vi "MegaAnalysis5.vi"() -> ()   [LabVIEW 2016] (continued)
                n2287 = property on="sampling freq" class="DigNum (strict)"() -> ("Value"=w5459:dbl)  [unwired: 2 in, 2 out]
                n2288 = property on="high cutoff" class="DigNum (strict)"() -> ("Value"=w5456:dbl)  [unwired: 2 in, 2 out]
                n2289 = property on="phase" class="DigNum (strict)"() -> ("Value"=w5444:dbl)  [unwired: 2 in, 2 out]
                n2290 = property on="phase" class="DigNum (strict)"() -> ("Value"=w5451:dbl)  [unwired: 2 in, 2 out]
                n2291 = property on="gamma" class="DigNum (strict)"() -> ("Value"=w5443:dbl)  [unwired: 2 in, 2 out]
                n2292 = property on="order" class="DigNum (strict)"() -> ("Value"=w5455:i32)  [unwired: 2 in, 2 out]
                n2293 = property on="poly sub" class="DigNum (strict)"() -> ("Value"=w5458:dbl)  [unwired: 2 in, 2 out]
                n2294 = Bundle("Value"=w5465, "Value"=w5464, "Value"=w5463, "Value"=w5462, "Value"=w5461, "Value"=w5460, "Value"=w5459, "Value"=w5458, "Value"=w5457, "Value"=w5456, "Value"=w5455, "Value"=w5454, "Value"=w5453, "Value"=w5452, "Value"=w5451, "Value"=w5450, "Value"=w5449, "Value"=w5448, "Value"=w5446, "Value"=w5445, "Value"=w5444, "Value"=w5443) -> (w5447:T37)  [unwired: 1 out]
              }
              frame #2 {
                n2295 = property class="Bool (strict)"() -> ("Value"=w5469:bool)  [unwired: 2 in, 2 out]
                n2296 = property on="cut off selection" class="Arr (strict)"() -> ("Value"=w5468:T10)  [unwired: 2 in, 2 out]
                n2297 = property on="window" class="Ring (strict)"() -> ("Value"=w5467:T9)  [unwired: 2 in, 2 out]
                n2298 = Bundle("Value"=w5469, "Value"=w5468, "Value"=w5467) -> (w5466:T38)  [unwired: 1 out]
              }
              frame #3 {
                n2299 = property on="append string onto file name" class="Str"() -> ("Value"=w5473:string)  [unwired: 2 in, 2 out]
                n2300 = property class="Bool (strict)"() -> ("Value"=w5474:bool)  [unwired: 2 in, 2 out]
                n2301 = property class="Bool (strict)"() -> ("Value"=w5472:bool)  [unwired: 2 in, 2 out]
                n2302 = property class="DigNum (strict)"() -> ("Value"=w5471:u8)  [unwired: 2 in, 2 out]
                n2303 = Bundle("Value"=w5474, "Value"=w5473, "Value"=w5472, "Value"=w5471) -> (w5470:T30)  [unwired: 1 out]
              }
              frame #4 {
                n2304 = property on="upper" class="DigNum (strict)"() -> ("Value"=w5478:dbl)  [unwired: 2 in, 2 out]
                n2305 = property class="Bool (strict)"() -> ("Value"=w5479:bool)  [unwired: 2 in, 2 out]
                n2306 = property on="append name" class="Str"() -> ("Value"=w5476:string)  [unwired: 2 in, 2 out]
                n2307 = property on="lower" class="DigNum (strict)"() -> ("Value"=w5477:dbl)  [unwired: 2 in, 2 out]
                n2308 = Bundle("Value"=w5479, "Value"=w5478, "Value"=w5477, "Value"=w5476) -> (w5475:T39)  [unwired: 1 out]
              }
              frame #5 {
                n2309 = Bundle(w5485, w5484, w5483, w5482, w5481) -> (w5480:T40)  [unwired: 1 out]
              }
            }
            n2310 = property class="Ring (strict)"() -> ("Value"=w5436:u16)  [unwired: 2 in, 2 out]
            n2311 = Bundle("Value"=w5436, w5435) -> (w5434:T41)  [unwired: 1 out]
          }
          frame #4 {
            n2312 = stacked-sequence {
              seq-local: [w5491 _ _] -> [_ _ w5504]
              seq-local: [_ w5498 _] -> [_ _ w5503]
              tunnel: [_ _ w5502] -> w5487
              frame #0 {
                n2313 = property on="spectrum type" class="Ring (strict)"() -> ("Value"=w5497:u16)  [unwired: 2 in, 2 out]
                n2314 = property on="interpolate in:" class="Ring (strict)"() -> ("Value"=w5496:u16)  [unwired: 2 in, 2 out]
                n2315 = property on="peak finder threshold" class="DigNum (strict)"() -> ("Value"=w5490:dbl)  [unwired: 2 in, 2 out]
                n2316 = property class="Bool (strict)"() -> ("Value"=w5495:bool)  [unwired: 2 in, 2 out]
                n2317 = property on="width" class="DigNum (strict)"() -> ("Value"=w5489:dbl)  [unwired: 2 in, 2 out]
                n2318 = property on="padding" class="Ring (strict)"() -> ("Value"=w5494:u16)  [unwired: 2 in, 2 out]
                n2319 = property on="truncate spectrum" class="Ring (strict)"() -> ("Value"=w5492:u16)  [unwired: 2 in, 2 out]
                n2320 = property on="Increase spectral density" class="Ring (strict)"() -> ("Value"=w5493:u16)  [unwired: 2 in, 2 out]
                n2321 = Bundle("Value"=w5497, "Value"=w5496, "Value"=w5495, "Value"=w5490, "Value"=w5494, "Value"=w5493, "Value"=w5492, "Value"=w5489) -> (w5491:T42)  [unwired: 1 out]
              }
              frame #1 {
                n2322 = property on="Maximum Entropy M" class="DigNum (strict)"() -> ("Value"=w5500:dbl)  [unwired: 2 in, 2 out]
                n2323 = property on="FT window" class="Ring (strict)"() -> ("Value"=w5501:T9)  [unwired: 2 in, 2 out]
                n2324 = property on="append name" class="Str"() -> ("Value"=w5499:string)  [unwired: 2 in, 2 out]
                n2325 = Bundle("Value"=w5501, "Value"=w5500, "Value"=w5499) -> (w5498:cluster{"Value":T9, "Value":dbl, "Value":string})  [unwired: 1 out]
              }
              frame #2 {
                n2326 = Bundle(w5504, w5503) -> (w5502:T43)  [unwired: 1 out]
              }
            }
            n2327 = property class="Ring (strict)"() -> ("Value"=w5488:u16)  [unwired: 2 in, 2 out]
            n2328 = Bundle("Value"=w5488, w5487) -> (w5486:T44)  [unwired: 1 out]
          }
          frame #5 {
            n2329 = stacked-sequence {
              seq-local: [w5509 _ _] -> [_ _ w5517]
              seq-local: [_ w5514 _] -> [_ _ w5516]
              tunnel: [_ _ w5515] -> w5505
              frame #0 {
                n2330 = property on="variable (T)" class="Arr (strict)"() -> ("Value"=w5513:dbl[])  [unwired: 2 in, 2 out]
                n2331 = property on="interpolation method" class="Ring (strict)"() -> ("Value"=w5506:i32)  [unwired: 2 in, 2 out]
                n2332 = property on="frequencies" class="Arr (strict)"() -> ("Value"=w5510:dbl[])  [unwired: 2 in, 2 out]
                n2333 = property class="Bool (strict)"() -> ("Value"=w5512:bool)  [unwired: 2 in, 2 out]
                n2334 = property on="points" class="DigNum (strict)"() -> ("Value"=w5511:u32)  [unwired: 2 in, 2 out]
                n2335 = property on="phase" class="DigNum (strict)"() -> ("Value"=w5507:dbl)  [unwired: 2 in, 2 out]
                n2336 = property on="amplitude" class="Ring (strict)"() -> ("Value"=w5508:u16)  [unwired: 2 in, 2 out]
                n2337 = Bundle("Value"=w5513, "Value"=w5512, "Value"=w5511, "Value"=w5510, "Value"=w5506, "Value"=w5508, "Value"=w5507) -> (w5509:T45)  [unwired: 1 out]
              }
              frame #1 {
                n2338 = property on="append name" class="Str"() -> ("Value"=w5514:string)  [unwired: 2 in, 2 out]
              }
              frame #2 {
                n2339 = Bundle(w5517, "Value"=w5516) -> (w5515:T46)  [unwired: 1 out]
              }
            }
          }
          frame #6 {
            n2340 = Bundle(w5529, w5528, w5527, w5526, w5525, w5524, "Notes (saved along with settings)"="Notes (saved along with settings)") -> (w5519:T47)  [unwired: 1 out]
            n2341 = To Variant(anything=w5519) -> (Variant=w5523:variant)
            n2342 = Variant To Flattened String(Variant=w5523) -> (data string=w5520:string, 1:w5522:i16[])
            n2343 = case shown="True" "?" {
              tunnel: w5520 -> [_ w5531]
              frame False {
              }
              frame True {
                n2344 = Write to Text File(prompt (Choose or enter file path)="Save current MegaAnalysis settings", text=w5531) -> ()  [unwired: 1 in, 4 out]
              }
            }
          }
          frame #7 {
            n2345 = case shown="True" w5534 {
              tunnel: w5533 -> [_ w5542]
              tunnel: w5532 -> [_ w5543]
              frame False {
              }
              frame True {
                n2346 = Read from Text File() -> (text=w5544:string)  [unwired: 1 in, 6 out]
                n2347 = Flattened String To Variant(6:w5544, 7:w5542) -> (3:w5545:variant)  [unwired: 1 in, 1 out]
                n2348 = Variant To Data(type=w5543, Variant=w5545) -> (data=w5546:T47)  [unwired: 1 in, 1 out]
                n2349 = Unbundle(w5546) -> (w5541:T19, w5540:T28, w5539:T35, w5538:T41, w5537:T44, w5536:T46, "Notes (saved along with settings)"=w5535:string)
                n2350 = stacked-sequence {
                  tunnel: w5541 -> [w5553 _ _ _ _ _]
                  tunnel: w5540 -> [_ w5554 _ _ _ _]
                  tunnel: w5539 -> [_ _ w5654 _ _ _]
                  tunnel: w5538 -> [_ _ _ w5706 _ _]
                  tunnel: w5537 -> [_ _ _ _ w5754 _]
                  tunnel: w5536 -> [_ _ _ _ _ w5776]
                  frame #0 {
                    n2351 = Unbundle(w5553) -> ("Value"=w5552:bool, "Value"=w5551:bool, "Value"=w5550:bool, "Value"=w5549:bool, "Value"=w5548:bool, "Value"=w5547:bool)
                    n2352 = property class="Bool (strict)"("Val(Sgnl)"=w5550) -> ()  [unwired: 2 in, 2 out]
                    n2353 = property class="Bool (strict)"("Val(Sgnl)"=w5549) -> ()  [unwired: 2 in, 2 out]
                    n2354 = property class="Bool (strict)"("Val(Sgnl)"=w5548) -> ()  [unwired: 2 in, 2 out]
                    n2355 = property class="Bool (strict)"("Val(Sgnl)"=w5551) -> ()  [unwired: 2 in, 2 out]
                    n2356 = property class="Bool (strict)"("Val(Sgnl)"=w5547) -> ()  [unwired: 2 in, 2 out]
                    n2357 = property class="Bool (strict)"("Val(Sgnl)"=w5552) -> ()  [unwired: 2 in, 2 out]
                  }
                  frame #1 {
                    n2358 = Unbundle(w5554) -> ("Value"=w5563:u16, "Value"=w5562:u16, "Value"=w5561:string, w5555:T27)
                    n2359 = property on="file format" class="Str"("Val(Sgnl)"=w5561) -> ()  [unwired: 2 in, 2 out]
                    n2360 = property class="Ring (strict)"("Val(Sgnl)"=w5563) -> ()  [unwired: 2 in, 2 out]
                    n2361 = property on="skip" class="DigNum (strict)"("Val(Sgnl)"=w5562) -> ()  [unwired: 2 in, 2 out]
                    n2362 = Unbundle(w5555) -> ("Value"=w5560:path[], w5559:T24, w5558:T25, w5557:T26, w5556:cluster{"Value":string, "Value":bool})
                    n2363 = stacked-sequence {
                      tunnel: w5560 -> [w5564 _ _ _ _]
                      tunnel: w5559 -> [_ w5572 _ _ _]
                      tunnel: w5558 -> [_ _ w5626 _ _]
                      tunnel: w5557 -> [_ _ _ w5642 _]
                      tunnel: w5556 -> [_ _ _ _ w5645]
                      frame #0 {
                        n2364 = property on="files to be imported" class="Arr (strict)"("Val(Sgnl)"=w5564) -> ()  [unwired: 2 in, 2 out]
                      }
                      frame #1 {
                        n2365 = Unbundle(w5572) -> ("Value"=w5571:u16, "Value"=w5570:bool, w5569:T20, w5568:T21, w5567:T22, w5566:T23, w5565:T23)
                        n2366 = property class="Bool (strict)"("Val(Sgnl)"=w5570) -> ()  [unwired: 2 in, 2 out]
                        n2367 = property on="column selection options (for each file)" class="Ring (strict)"("Val(Sgnl)"=w5571) -> ()  [unwired: 2 in, 2 out]
                        n2368 = stacked-sequence {
                          tunnel: w5569 -> [w5577 _ _ _ _]
                          tunnel: w5568 -> [_ w5582 _ _ _]
                          tunnel: w5567 -> [_ _ w5595 _ _]
                          tunnel: w5566 -> [_ _ _ w5605 _]
                          tunnel: w5565 -> [_ _ _ _ w5615]
                          frame #0 {
                            n2369 = Unbundle(w5577) -> ("Value"=w5576:u16, "Value"=w5575:dbl, "Value"=w5574:u16[], "Value"=w5573:ext[])
                            n2370 = property on="time column selection" class="Arr (strict)"("Val(Sgnl)"=w5574) -> ()  [unwired: 2 in, 2 out]
                            n2371 = property on="time column rescale" class="Arr (strict)"("Val(Sgnl)"=w5573) -> ()  [unwired: 2 in, 2 out]
                            n2372 = property on="option" class="Ring (strict)"("Val(Sgnl)"=w5576) -> ()  [unwired: 2 in, 2 out]
                            n2373 = property on="time interval  (for series)" class="DigNum (strict)"("Val(Sgnl)"=w5575) -> ()  [unwired: 2 in, 2 out]
                          }
                          frame #1 {
                            n2374 = Unbundle(w5582) -> ("Value"=w5581:u16, "Value"=w5580:u16[], "Value"=w5579:ext[], "Value"=w5578:bool)
                            n2375 = property class="Bool (strict)"("Val(Sgnl)"=w5578) -> ()  [unwired: 2 in, 2 out]
                            n2376 = property on="option" class="Ring (strict)"("Val(Sgnl)"=w5581) -> ()  [unwired: 2 in, 2 out]
                            n2377 = property on="dB/dt column selection" class="Arr (strict)"("Val(Sgnl)"=w5580) -> ()  [unwired: 2 in, 2 out]
                            n2378 = property on="dB/dt column rescale" class="Arr (strict)"("Val(Sgnl)"=w5579) -> ()  [unwired: 2 in, 2 out]
                          }
                          frame #2 {
                            n2379 = Unbundle(w5595) -> ("Value"=w5594:u16, "Value"=w5593:dbl, "B column selection"=w5583:u16[], "Value"=w5592:ext[], "Value"=w5591:ext[], "Value"=w5590:ext[], "Value"=w5589:bool, "Value"=w5588:bool, "Value"=w5587:bool, "Value"=w5586:bool, "Value"=w5585:u32, "Value"=w5584:dbl)
                            n2380 = property class="DigNum (strict)"("Val(Sgnl)"=w5585) -> ()  [unwired: 2 in, 2 out]
                            n2381 = property class="DigNum (strict)"("Val(Sgnl)"=w5584) -> ()  [unwired: 2 in, 2 out]
                            n2382 = property on="B column rescale" class="Arr (strict)"("Val(Sgnl)"=w5592) -> ()  [unwired: 2 in, 2 out]
                            n2383 = property on="angle theta (cos theta renorm.)" class="Arr (strict)"("Val(Sgnl)"=w5591) -> ()  [unwired: 2 in, 2 out]
                            n2384 = local write "B column selection"(w5583) -> ()
                            n2385 = property on="B column offset" class="Arr (strict)"("Val(Sgnl)"=w5590) -> ()  [unwired: 2 in, 2 out]
                            n2386 = property on="option" class="Ring (strict)"("Val(Sgnl)"=w5594) -> ()  [unwired: 2 in, 2 out]
                            n2387 = property on="pretrigger time for integration" class="DigNum (strict)"("Val(Sgnl)"=w5593) -> ()  [unwired: 2 in, 2 out]
                            n2388 = property class="Bool (strict)"("Val(Sgnl)"=w5587) -> ()  [unwired: 2 in, 2 out]
                            n2389 = property class="Bool (strict)"("Val(Sgnl)"=w5586) -> ()  [unwired: 2 in, 2 out]
                            n2390 = property class="Bool (strict)"("Val(Sgnl)"=w5588) -> ()  [unwired: 2 in, 2 out]
                            n2391 = property class="Bool (strict)"("Val(Sgnl)"=w5589) -> ()  [unwired: 2 in, 2 out]
                          }
                          frame #3 {
                            n2392 = Unbundle(w5605) -> ("Value"=w5604:u16, "Value"=w5603:dbl, "Value"=w5602:bool, "Value"=w5600:i64, "Value"=w5601:u16[], "Value"=w5599:ext[], "Value"=w5598:ext[], "Value"=w5597:bool, "Value"=w5596:bool)
                            n2393 = property on="data column offset" class="Arr (strict)"("Val(Sgnl)"=w5598) -> ()  [unwired: 2 in, 2 out]
                            n2394 = property on="data column selection" class="Arr (strict)"("Val(Sgnl)"=w5601) -> ()  [unwired: 2 in, 2 out]
                            n2395 = property on="data column rescale" class="Arr (strict)"("Val(Sgnl)"=w5599) -> ()  [unwired: 2 in, 2 out]
                            n2396 = property on="option" class="Ring (strict)"("Val(Sgnl)"=w5604) -> ()  [unwired: 2 in, 2 out]
                            n2397 = property on="pretrigger time for integration" class="DigNum (strict)"("Val(Sgnl)"=w5603) -> ()  [unwired: 2 in, 2 out]
                            n2398 = property class="Bool (strict)"("Val(Sgnl)"=w5602) -> ()  [unwired: 2 in, 2 out]
                            n2399 = property class="Bool (strict)"("Val(Sgnl)"=w5597) -> ()  [unwired: 2 in, 2 out]
                            n2400 = property class="Bool (strict)"("Val(Sgnl)"=w5596) -> ()  [unwired: 2 in, 2 out]
                            n2401 = property class="DigNum (strict)"("Val(Sgnl)"=w5600) -> ()  [unwired: 2 in, 2 out]
                          }
                          frame #4 {
                            n2402 = Unbundle(w5615) -> ("Value"=w5614:u16, "Value"=w5613:dbl, "Value"=w5612:bool, "Value"=w5611:i64, "Value"=w5610:u16[], "Value"=w5609:ext[], "Value"=w5608:ext[], "Value"=w5607:bool, "Value"=w5606:bool)
                            n2403 = property on="option" class="Ring (strict)"("Val(Sgnl)"=w5614) -> ()  [unwired: 2 in, 2 out]
                            n2404 = property on="data column rescale" class="Arr (strict)"("Val(Sgnl)"=w5609) -> ()  [unwired: 2 in, 2 out]
                            n2405 = property on="data column selection" class="Arr (strict)"("Val(Sgnl)"=w5610) -> ()  [unwired: 2 in, 2 out]
                            n2406 = property on="data column offset" class="Arr (strict)"("Val(Sgnl)"=w5608) -> ()  [unwired: 2 in, 2 out]
                            n2407 = property on="pretrigger time for integration" class="DigNum (strict)"("Val(Sgnl)"=w5613) -> ()  [unwired: 2 in, 2 out]
                            n2408 = property class="Bool (strict)"("Val(Sgnl)"=w5612) -> ()  [unwired: 2 in, 2 out]
                            n2409 = property class="Bool (strict)"("Val(Sgnl)"=w5606) -> ()  [unwired: 2 in, 2 out]
                            n2410 = property class="Bool (strict)"("Val(Sgnl)"=w5607) -> ()  [unwired: 2 in, 2 out]
                            n2411 = property class="DigNum (strict)"("Val(Sgnl)"=w5611) -> ()  [unwired: 2 in, 2 out]
                          }
                        }
                      }
                      frame #2 {
                        n2412 = Unbundle(w5626) -> ("Value"=w5625:bool, "Value"=w5624:bool, "Value"=w5623:bool, "Value"=w5622:u64, "Value"=w5621:ext, "Value"=w5620:ext, "Value"=w5619:u64, "Value"=w5618:ext, "Value"=w5617:ext, "Value"=w5616:bool)
                        n2413 = property class="Bool (strict)"("Val(Sgnl)"=w5625) -> ()  [unwired: 2 in, 2 out]
                        n2414 = property class="Bool (strict)"("Val(Sgnl)"=w5624) -> ()  [unwired: 2 in, 2 out]
                        n2415 = property class="Bool (strict)"("Val(Sgnl)"=w5623) -> ()  [unwired: 2 in, 2 out]
                        n2416 = property on="lower cutoff" class="DigNum (strict)"("Val(Sgnl)"=w5622) -> ()  [unwired: 2 in, 2 out]
                        n2417 = property on="lower cutoff" class="DigNum (strict)"("Val(Sgnl)"=w5621) -> ()  [unwired: 2 in, 2 out]
                        n2418 = property on="lower cutoff" class="DigNum (strict)"("Val(Sgnl)"=w5620) -> ()  [unwired: 2 in, 2 out]
                        n2419 = property class="Bool (strict)"("Val(Sgnl)"=w5616) -> ()  [unwired: 2 in, 2 out]
                        n2420 = property on="upper cutoff" class="DigNum (strict)"("Val(Sgnl)"=w5618) -> ()  [unwired: 2 in, 2 out]
                        n2421 = property on="upper cutoff" class="DigNum (strict)"("Val(Sgnl)"=w5619) -> ()  [unwired: 2 in, 2 out]
                        n2422 = property on="upper cutoff" class="DigNum (strict)"("Val(Sgnl)"=w5617) -> ()  [unwired: 2 in, 2 out]
                      }
                      frame #3 {
                        n2423 = Unbundle(w5642) -> ("Value"=w5641:u16, "Value"=w5640:u16, "Value"=w5639:dbl[], "Value"=w5638:T5, "Value"=w5637:dbl, "Value"=w5636:dbl, "Value"=w5635:i32, "Value"=w5634:dbl, "Value"=w5633:dbl, "Value"=w5632:dbl, "Value"=w5630:i32, "Value"=w5629:i32, "Value"=w5628:i32, "Value"=w5627:i32, "Value"=w5631:dbl)
                        n2424 = property on="filter selection" class="Ring (strict)"("Val(Sgnl)"=w5641) -> ()  [unwired: 2 in, 2 out]
                        n2425 = property on="sampling frequency option" class="Ring (strict)"("Val(Sgnl)"=w5640) -> ()  [unwired: 2 in, 2 out]
                        n2426 = property on="sampling frequency" class="Arr (strict)"("Val(Sgnl)"=w5639) -> ()  [unwired: 2 in, 2 out]
                        n2427 = property on="passband ripple (dB)" class="DigNum (strict)"("Val(Sgnl)"=w5632) -> ()  [unwired: 2 in, 2 out]
                        n2428 = property on="filter type" class="Enum (strict)"("Val(Sgnl)"=w5638) -> ()  [unwired: 2 in, 2 out]
                        n2429 = property on="order" class="DigNum (strict)"("Val(Sgnl)"=w5635) -> ()  [unwired: 2 in, 2 out]
                        n2430 = property on="window" class="Ring (strict)"("Val(Sgnl)"=w5630) -> ()  [unwired: 2 in, 2 out]
                        n2431 = property on="left rank" class="DigNum (strict)"("Val(Sgnl)"=w5628) -> ()  [unwired: 2 in, 2 out]
                        n2432 = property on="low cutoff freq: fl" class="DigNum (strict)"("Val(Sgnl)"=w5637) -> ()  [unwired: 2 in, 2 out]
                        n2433 = property on="ripple(dB)" class="DigNum (strict)"("Val(Sgnl)"=w5634) -> ()  [unwired: 2 in, 2 out]
                        n2434 = property on="stopband attenuation (dB)" class="DigNum (strict)"("Val(Sgnl)"=w5631) -> ()  [unwired: 2 in, 2 out]
                        n2435 = property on="right rank" class="DigNum (strict)"("Val(Sgnl)"=w5627) -> ()  [unwired: 2 in, 2 out]
                        n2436 = property on="taps" class="DigNum (strict)"("Val(Sgnl)"=w5629) -> ()  [unwired: 2 in, 2 out]
                        n2437 = property on="attenuation (dB)" class="DigNum (strict)"("Val(Sgnl)"=w5633) -> ()  [unwired: 2 in, 2 out]
                        n2438 = property on="high cutoff freq: fh" class="DigNum (strict)"("Val(Sgnl)"=w5636) -> ()  [unwired: 2 in, 2 out]
                      }
                      frame #4 {
                        n2439 = Unbundle(w5645) -> ("Value"=w5644:string, "Value"=w5643:bool)
                        n2440 = property class="Bool (strict)"("Val(Sgnl)"=w5643) -> ()  [unwired: 2 in, 2 out]
                        n2441 = property on="append name" class="Str"("Val(Sgnl)"=w5644) -> ()  [unwired: 2 in, 2 out]
                      }
                    }
                  }
                  frame #2 {
                    n2442 = Unbundle(w5654) -> ("Value"=w5653:u16, w5652:T34)
                    n2443 = property class="Ring (strict)"("Val(Sgnl)"=w5653) -> ()  [unwired: 2 in, 2 out]
                    n2444 = Unbundle(w5652) -> (w5651:T29, w5650:T30, w5649:T31, w5648:T32, "Value"=w5647:string, w5646:T33)
                    n2445 = stacked-sequence {
                      tunnel: w5651 -> [w5659 _ _ _ _ _]
                      tunnel: w5650 -> [_ w5664 _ _ _ _]
                      tunnel: w5649 -> [_ _ w5676 _ _ _]
                      tunnel: w5648 -> [_ _ _ w5691 _ _]
                      tunnel: w5647 -> [_ _ _ _ _ w5698]
                      tunnel: w5646 -> [_ _ _ _ w5697 _]
                      frame #0 {
                        n2446 = Unbundle(w5659) -> ("Value"=w5658:bool, "Value"=w5657:u16, "Value"=w5656:u16, "Value"=w5655:u8)
                        n2447 = property on="reference option" class="Ring (strict)"("Val(Sgnl)"=w5657) -> ()  [unwired: 2 in, 2 out]
                        n2448 = property class="Bool (strict)"("Val(Sgnl)"=w5658) -> ()  [unwired: 2 in, 2 out]
                        n2449 = property on="file name options" class="Ring (strict)"("Val(Sgnl)"=w5656) -> ()  [unwired: 2 in, 2 out]
                        n2450 = property class="DigNum (strict)"("Val(Sgnl)"=w5655) -> ()  [unwired: 2 in, 2 out]
                      }
                      frame #1 {
                        n2451 = Unbundle(w5664) -> ("Value"=w5663:bool, "Value"=w5662:string, "Value"=w5661:bool, "Value"=w5660:u8)
                        n2452 = property class="Bool (strict)"("Val(Sgnl)"=w5663) -> ()  [unwired: 2 in, 2 out]
                        n2453 = property on="append string onto file name" class="Str"("Val(Sgnl)"=w5662) -> ()  [unwired: 2 in, 2 out]
                        n2454 = property class="Bool (strict)"("Val(Sgnl)"=w5661) -> ()  [unwired: 2 in, 2 out]
                        n2455 = property class="DigNum (strict)"("Val(Sgnl)"=w5660) -> ()  [unwired: 2 in, 2 out]
                      }
                      frame #2 {
                        n2456 = Unbundle(w5676) -> ("Value"=w5675:u16, "Value"=w5674:bool, "Value"=w5673:dbl, "Value"=w5672:bool, "Value"=w5671:dbl, "Value"=w5670:bool, "Value"=w5669:dbl, "Value"=w5668:bool, "Value"=w5667:dbl, "Value"=w5666:bool, "Value"=w5665:dbl)
                        n2457 = property on="data options" class="Ring (strict)"("Val(Sgnl)"=w5675) -> ()  [unwired: 2 in, 2 out]
                        n2458 = property class="Bool (strict)"("Val(Sgnl)"=w5674) -> ()  [unwired: 2 in, 2 out]
                        n2459 = property class="Bool (strict)"("Val(Sgnl)"=w5670) -> ()  [unwired: 2 in, 2 out]
                        n2460 = property class="Bool (strict)"("Val(Sgnl)"=w5672) -> ()  [unwired: 2 in, 2 out]
                        n2461 = property class="Bool (strict)"("Val(Sgnl)"=w5668) -> ()  [unwired: 2 in, 2 out]
                        n2462 = property class="Bool (strict)"("Val(Sgnl)"=w5666) -> ()  [unwired: 2 in, 2 out]
                        n2463 = property class="DigNum (strict)"("Val(Sgnl)"=w5673) -> ()  [unwired: 2 in, 2 out]
                        n2464 = property class="DigNum (strict)"("Val(Sgnl)"=w5665) -> ()  [unwired: 2 in, 2 out]
                        n2465 = property class="DigNum (strict)"("Val(Sgnl)"=w5667) -> ()  [unwired: 2 in, 2 out]
                        n2466 = property class="DigNum (strict)"("Val(Sgnl)"=w5669) -> ()  [unwired: 2 in, 2 out]
                        n2467 = property class="DigNum (strict)"("Val(Sgnl)"=w5671) -> ()  [unwired: 2 in, 2 out]
                      }
                      frame #3 {
                        n2468 = Unbundle(w5691) -> ("Value"=w5690:bool, "Value"=w5689:dbl, "Value"=w5677:u16, "Value"=w5688:cluster{dbl, "and":dbl}[], "Value"=w5687:bool, "Value"=w5686:dbl, "Value"=w5685:dbl, "Value"=w5684:bool, "Value"=w5683:dbl[][], "Value"=w5682:dbl[][], "Value"=w5681:dbl[], "Value"=w5680:dbl[], "Value"=w5679:dbl, "Value"=w5678:dbl)
                        n2469 = property on="row" class="Arr (strict)"("Val(Sgnl)"=w5683) -> ()  [unwired: 2 in, 2 out]
                        n2470 = property on="threshold # of points below which field variations are ignored" class="DigNum (strict)"("Val(Sgnl)"=w5686) -> ()  [unwired: 2 in, 2 out]
                        n2471 = property on="field limits:" class="Ring (strict)"("Val(Sgnl)"=w5677) -> ()  [unwired: 2 in, 2 out]
                        n2472 = property class="Bool (strict)"("Val(Sgnl)"=w5690) -> ()  [unwired: 2 in, 2 out]
                        n2473 = property on="maxima above:" class="DigNum (strict)"("Val(Sgnl)"=w5679) -> ()  [unwired: 2 in, 2 out]
                        n2474 = property on="fields" class="Arr (strict)"("Val(Sgnl)"=w5682) -> ()  [unwired: 2 in, 2 out]
                        n2475 = property on="(slow on large data sets but good for treating small fluctuations in field)" class="DigNum (strict)"("Val(Sgnl)"=w5689) -> ()  [unwired: 2 in, 2 out]
                        n2476 = property class="Arr (strict)"("Val(Sgnl)"=w5688) -> ()  [unwired: 2 in, 2 out]
                        n2477 = property on="consider variations in B field only above:" class="DigNum (strict)"("Val(Sgnl)"=w5685) -> ()  [unwired: 2 in, 2 out]
                        n2478 = property on="rising sweep start index" class="Arr (strict)"("Val(Sgnl)"=w5681) -> ()  [unwired: 2 in, 2 out]
                        n2479 = property class="Bool (strict)"("Val(Sgnl)"=w5687) -> ()  [unwired: 2 in, 2 out]
                        n2480 = property on="minima below :" class="DigNum (strict)"("Val(Sgnl)"=w5678) -> ()  [unwired: 2 in, 2 out]
                        n2481 = property class="Bool (strict)"("Val(Sgnl)"=w5684) -> ()  [unwired: 2 in, 2 out]
                        n2482 = property on="falling sweep start index" class="Arr (strict)"("Val(Sgnl)"=w5680) -> ()  [unwired: 2 in, 2 out]
                      }
                      frame #4 {
                        n2483 = Unbundle(w5697) -> ("Value"=w5696:u16, "Value"=w5695:u8, "Value"=w5694:u16, "Value"=w5693:dbl, "Value"=w5692:dbl)
                        n2484 = property on="offset options" class="Ring (strict)"("Val(Sgnl)"=w5694) -> ()  [unwired: 2 in, 2 out]
                        n2485 = property on="field smoothing" class="Ring (strict)"("Val(Sgnl)"=w5696) -> ()  [unwired: 2 in, 2 out]
                        n2486 = property on="offset value" class="DigNum (strict)"("Val(Sgnl)"=w5693) -> ()  [unwired: 2 in, 2 out]
                        n2487 = property on="smoothing ratio (must be appreciably larger than 1)" class="DigNum (strict)"("Val(Sgnl)"=w5695) -> ()  [unwired: 2 in, 2 out]
                        n2488 = property on="sweeprate-dependent  offset multiplier" class="DigNum (strict)"("Val(Sgnl)"=w5692) -> ()  [unwired: 2 in, 2 out]
                      }
                      frame #5 {
                        n2489 = property on="append name" class="Str"("Val(Sgnl)"=w5698) -> ()  [unwired: 2 in, 2 out]
                      }
                    }
                  }
                  frame #3 {
                    n2490 = Unbundle(w5706) -> ("Value"=w5705:u16, w5704:T40)
                    n2491 = property class="Ring (strict)"("Val(Sgnl)"=w5705) -> ()  [unwired: 2 in, 2 out]
                    n2492 = Unbundle(w5704) -> (w5703:T36, w5702:T37, w5701:T38, w5700:T30, w5699:T39)
                    n2493 = stacked-sequence {
                      tunnel: w5703 -> [w5712 _ _ _ _]
                      tunnel: w5702 -> [_ w5735 _ _ _]
                      tunnel: w5701 -> [_ _ w5739 _ _]
                      tunnel: w5700 -> [_ _ _ w5744 _]
                      tunnel: w5699 -> [_ _ _ _ w5749]
                      frame #0 {
                        n2494 = Unbundle(w5712) -> ("Value"=w5711:u16, "Value"=w5710:u64, "Value"=w5709:i32, "Value"=w5708:u16, "Value"=w5707:bool)
                        n2495 = property on="interpolate in:" class="Ring (strict)"("Val(Sgnl)"=w5711) -> ()  [unwired: 2 in, 2 out]
                        n2496 = property on="rising and falling field options" class="Ring (strict)"("Val(Sgnl)"=w5708) -> ()  [unwired: 2 in, 2 out]
                        n2497 = property class="Bool (strict)"("Val(Sgnl)"=w5707) -> ()  [unwired: 2 in, 2 out]
                        n2498 = property on="# points" class="DigNum (strict)"("Val(Sgnl)"=w5710) -> ()  [unwired: 2 in, 2 out]
                        n2499 = property on="method" class="Ring (strict)"("Val(Sgnl)"=w5709) -> ()  [unwired: 2 in, 2 out]
                      }
                      frame #1 {
                        n2500 = Unbundle(w5735) -> ("Value"=w5734:u16, "Value"=w5733:u16, "Value"=w5732:u16, "Value"=w5731:u16, "Value"=w5730:bool, "Value"=w5729:T5, "Value"=w5728:dbl, "Value"=w5727:dbl, "Value"=w5726:dbl, "Value"=w5725:dbl, "Value"=w5724:i32, "Value"=w5723:dbl, "Value"=w5722:dbl, "Value"=w5721:dbl, "Value"=w5720:dbl, "Value"=w5719:T8, "Value"=w5718:u8, "Value"=w5717:dbl, "Value"=w5716:dbl, "Value"=w5715:dbl, "Value"=w5714:dbl, "Value"=w5713:dbl)
                        n2501 = property on="gamma" class="DigNum (strict)"("Val(Sgnl)"=w5717) -> ()  [unwired: 2 in, 2 out]
                        n2502 = property on="special background/filter operations" class="Ring (strict)"("Val(Sgnl)"=w5734) -> ()  [unwired: 2 in, 2 out]
                        n2503 = property class="Bool (strict)"("Val(Sgnl)"=w5730) -> ()  [unwired: 2 in, 2 out]
                        n2504 = property on="background subtraction method" class="Ring (strict)"("Val(Sgnl)"=w5733) -> ()  [unwired: 2 in, 2 out]
                        n2505 = property on="low cutoff" class="DigNum (strict)"("Val(Sgnl)"=w5726) -> ()  [unwired: 2 in, 2 out]
                        n2506 = property on="filter type" class="Enum (strict)"("Val(Sgnl)"=w5729) -> ()  [unwired: 2 in, 2 out]
                        n2507 = property on="algorithm" class="Enum (strict)"("Val(Sgnl)"=w5719) -> ()  [unwired: 2 in, 2 out]
                        n2508 = property on="F" class="DigNum (strict)"("Val(Sgnl)"=w5723) -> ()  [unwired: 2 in, 2 out]
                        n2509 = property on="subtraction type" class="Ring (strict)"("Val(Sgnl)"=w5732) -> ()  [unwired: 2 in, 2 out]
                        n2510 = property on="sampling freq" class="DigNum (strict)"("Val(Sgnl)"=w5728) -> ()  [unwired: 2 in, 2 out]
                        n2511 = property on="high cutoff" class="DigNum (strict)"("Val(Sgnl)"=w5725) -> ()  [unwired: 2 in, 2 out]
                        n2512 = property on="amp" class="DigNum (strict)"("Val(Sgnl)"=w5722) -> ()  [unwired: 2 in, 2 out]
                        n2513 = property on="polynomial order" class="DigNum (strict)"("Val(Sgnl)"=w5718) -> ()  [unwired: 2 in, 2 out]
                        n2514 = property on="post interp amplitude/field modifier" class="Ring (strict)"("Val(Sgnl)"=w5731) -> ()  [unwired: 2 in, 2 out]
                        n2515 = property on="gamma" class="DigNum (strict)"("Val(Sgnl)"=w5721) -> ()  [unwired: 2 in, 2 out]
                        n2516 = property on="poly sub" class="DigNum (strict)"("Val(Sgnl)"=w5727) -> ()  [unwired: 2 in, 2 out]
                        n2517 = property on="order" class="DigNum (strict)"("Val(Sgnl)"=w5724) -> ()  [unwired: 2 in, 2 out]
                        n2518 = property on="f" class="DigNum (strict)"("Val(Sgnl)"=w5716) -> ()  [unwired: 2 in, 2 out]
                        n2519 = property on="phase" class="DigNum (strict)"("Val(Sgnl)"=w5720) -> ()  [unwired: 2 in, 2 out]
                        n2520 = property on="amp" class="DigNum (strict)"("Val(Sgnl)"=w5715) -> ()  [unwired: 2 in, 2 out]
                        n2521 = property on="phase" class="DigNum (strict)"("Val(Sgnl)"=w5714) -> ()  [unwired: 2 in, 2 out]
                        n2522 = property on="gamma" class="DigNum (strict)"("Val(Sgnl)"=w5713) -> ()  [unwired: 2 in, 2 out]
                      }
                      frame #2 {
                        n2523 = Unbundle(w5739) -> ("Value"=w5738:bool, "Value"=w5737:T10, "Value"=w5736:T9)
                        n2524 = property on="cut off selection" class="Arr (strict)"("Val(Sgnl)"=w5737) -> ()  [unwired: 2 in, 2 out]
                        n2525 = property class="Bool (strict)"("Val(Sgnl)"=w5738) -> ()  [unwired: 2 in, 2 out]
                        n2526 = property on="window" class="Ring (strict)"("Val(Sgnl)"=w5736) -> ()  [unwired: 2 in, 2 out]
                      }
                      frame #3 {
                        n2527 = Unbundle(w5744) -> ("Value"=w5743:bool, "Value"=w5742:string, "Value"=w5741:bool, "Value"=w5740:u8)
                        n2528 = property class="Bool (strict)"("Val(Sgnl)"=w5741) -> ()  [unwired: 2 in, 2 out]
                        n2529 = property class="Bool (strict)"("Val(Sgnl)"=w5743) -> ()  [unwired: 2 in, 2 out]
                        n2530 = property on="append string onto file name" class="Str"("Val(Sgnl)"=w5742) -> ()  [unwired: 2 in, 2 out]
                        n2531 = property class="DigNum (strict)"("Val(Sgnl)"=w5740) -> ()  [unwired: 2 in, 2 out]
                      }
                      frame #4 {
                        n2532 = Unbundle(w5749) -> ("Value"=w5748:bool, "Value"=w5747:dbl, "Value"=w5746:dbl, "Value"=w5745:string)
                        n2533 = property on="append name" class="Str"("Val(Sgnl)"=w5745) -> ()  [unwired: 2 in, 2 out]
                        n2534 = property on="upper" class="DigNum (strict)"("Val(Sgnl)"=w5747) -> ()  [unwired: 2 in, 2 out]
                        n2535 = property class="Bool (strict)"("Val(Sgnl)"=w5748) -> ()  [unwired: 2 in, 2 out]
                        n2536 = property on="lower" class="DigNum (strict)"("Val(Sgnl)"=w5746) -> ()  [unwired: 2 in, 2 out]
                      }
                    }
                  }
                  frame #4 {
                    n2537 = Unbundle(w5754) -> ("Value"=w5753:u16, w5752:T43)
                    n2538 = property class="Ring (strict)"("Val(Sgnl)"=w5753) -> ()  [unwired: 2 in, 2 out]
                    n2539 = Unbundle(w5752) -> (w5751:T42, w5750:cluster{"Value":T9, "Value":dbl, "Value":string})
                    n2540 = stacked-sequence {
                      tunnel: w5751 -> [w5763 _]
                      tunnel: w5750 -> [_ w5767]
                      frame #0 {
                        n2541 = Unbundle(w5763) -> ("Value"=w5762:u16, "Value"=w5761:u16, "Value"=w5760:bool, "Value"=w5759:dbl, "Value"=w5757:u16, "Value"=w5756:u16, "Value"=w5755:u16, "Value"=w5758:dbl)
                        n2542 = property on="width" class="DigNum (strict)"("Val(Sgnl)"=w5758) -> ()  [unwired: 2 in, 2 out]
                        n2543 = property on="peak finder threshold" class="DigNum (strict)"("Val(Sgnl)"=w5759) -> ()  [unwired: 2 in, 2 out]
                        n2544 = property class="Bool (strict)"("Val(Sgnl)"=w5760) -> ()  [unwired: 2 in, 2 out]
                        n2545 = property on="spectrum type" class="Ring (strict)"("Val(Sgnl)"=w5762) -> ()  [unwired: 2 in, 2 out]
                        n2546 = property on="interpolate in:" class="Ring (strict)"("Val(Sgnl)"=w5761) -> ()  [unwired: 2 in, 2 out]
                        n2547 = property on="truncate spectrum" class="Ring (strict)"("Val(Sgnl)"=w5756) -> ()  [unwired: 2 in, 2 out]
                        n2548 = property on="padding" class="Ring (strict)"("Val(Sgnl)"=w5757) -> ()  [unwired: 2 in, 2 out]
                        n2549 = property on="Increase spectral density" class="Ring (strict)"("Val(Sgnl)"=w5755) -> ()  [unwired: 2 in, 2 out]
                      }
                      frame #1 {
                        n2550 = Unbundle(w5767) -> ("Value"=w5766:T9, "Value"=w5765:dbl, "Value"=w5764:string)
                        n2551 = property on="append name" class="Str"("Val(Sgnl)"=w5764) -> ()  [unwired: 2 in, 2 out]
                        n2552 = property on="Maximum Entropy M" class="DigNum (strict)"("Val(Sgnl)"=w5765) -> ()  [unwired: 2 in, 2 out]
                        n2553 = property on="FT window" class="Ring (strict)"("Val(Sgnl)"=w5766) -> ()  [unwired: 2 in, 2 out]
                      }
                    }
                  }
                  frame #5 {
                    n2554 = Unbundle(w5776) -> (w5775:T45)  [unwired: 1 out]
                    n2555 = Unbundle(w5775) -> ("Value"=w5774:dbl[], "Value"=w5773:bool, "Value"=w5771:u32, "Value"=w5772:dbl[], "Value"=w5770:i32, "Value"=w5769:u16, "Value"=w5768:dbl)
                    n2556 = property on="variable (T)" class="Arr (strict)"("Val(Sgnl)"=w5774) -> ()  [unwired: 2 in, 2 out]
                    n2557 = property on="interpolation method" class="Ring (strict)"("Val(Sgnl)"=w5770) -> ()  [unwired: 2 in, 2 out]
                    n2558 = property class="Bool (strict)"("Val(Sgnl)"=w5773) -> ()  [unwired: 2 in, 2 out]
                    n2559 = property on="amplitude" class="Ring (strict)"("Val(Sgnl)"=w5769) -> ()  [unwired: 2 in, 2 out]
                    n2560 = property on="phase" class="DigNum (strict)"("Val(Sgnl)"=w5768) -> ()  [unwired: 2 in, 2 out]
                    n2561 = property on="frequencies" class="Arr (strict)"("Val(Sgnl)"=w5772) -> ()  [unwired: 2 in, 2 out]
                    n2562 = property on="points" class="DigNum (strict)"("Val(Sgnl)"=w5771) -> ()  [unwired: 2 in, 2 out]
                  }
                }
                n2563 = property on="Notes (saved along with settings)" class="Str"("Val(Sgnl)"=w5535) -> ()  [unwired: 2 in, 2 out]
              }
            }
          }
        }
      }
      frame #10 {
        n2564 = Wait For Front Panel Activity() -> (0:w5779:u32)  [unwired: 3 out]
        n2565 = global write "status.vi" "String"("idle") -> ()
        n2566 = Stop(stop? (T)="?") -> ()
      }
    }
  }
